vi "Create Sweep.vi"(6 "Post action (indexing priority)":T1=[enum."Do Nothing", enum."Wait", enum."Do Nothing", enum."Do Nothing"], 8 "error in (no error)":errorcluster, 9 "Scan parameters":T3=[{"DAQ Channel"=2, "Label"="\nscaledVsg1=", "Start"=0.14, "End"=-0.060000000000000005, "Step"=-0.060000000000000005, "Rate"=0.0, "VISA resource name"=""}, {"DAQ Channel"=2, "Label"="\nscaledVsg1=", "Start"=0.14, "End"=-0.060000000000000005, "Step"=-0.060000000000000005, "Rate"=0.0, "VISA resource name"=""}, {"DAQ Channel"=2, "Label"="\nscaledVsg1=", "Start"=0.14, "End"=-0.060000000000000005, "Step"=-0.060000000000000005, "Rate"=0.0, "VISA resource name"=""}, {"DAQ Channel"=3, "Label"="\nscaledVsg1=", "Start"=0.14, "End"=-0.060000000000000005, "Step"=-0.060000000000000005, "Rate"=0.0, "VISA resource name"=""}] {"Rate" format="%.2f"; "Step" format="%#_6p"; "End" format="%#_6p"; "Start" format="%#_6p"}, 10 "Scan control":T5=[{"Priority"=enum."Priority 1", "Scan name"=enum."DSA_Vamp"}, {"Priority"=enum."Priority 2", "Scan name"=enum."DSA_Vsg1"}, {"Priority"=enum."Priority 0", "Scan name"=enum."DSA_Vsg2"}, {"Priority"=enum."Priority 2", "Scan name"=enum."DSA_Vsg3"}], 11 "SweepControl":refnum<class "SweepControl.lvclass">) -> (0 "error out":errorcluster, 3 "SweepControl":refnum<class "SweepControl.lvclass">)   [LabVIEW 2016, in "SweepControl.lvclass"]
uses:
  SweepControl.lvclass
  Typedefs/ScanControl.ctl
  Typedefs/Cluster - ScanControl.ctl
  Typedefs/Enum - Priority.ctl
  Typedefs/Enum - Action.ctl
  Typedefs/ScanParamters.ctl
  Typedefs/Cluster - ScanParamters.ctl
  Typedefs/PostAction.ctl
  Typedefs/Enum - PostAction.ctl
  SweepControl.lvclass/SweepControl.ctl
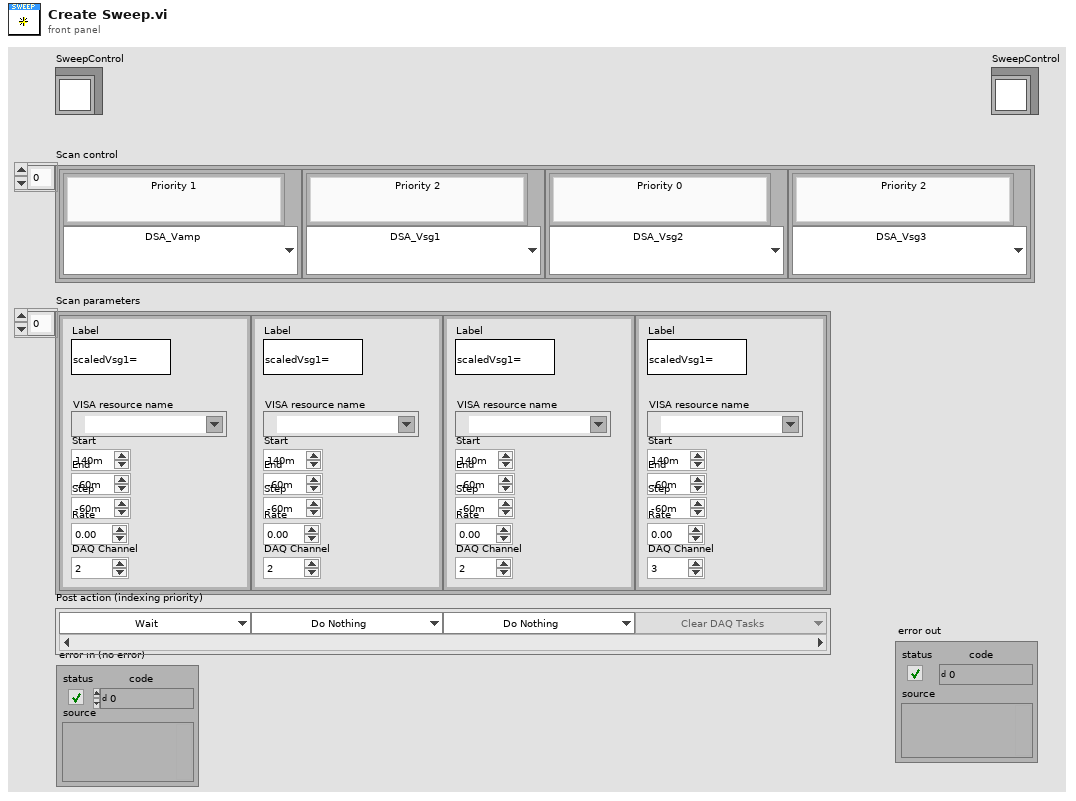
[diagram p1: front panel]
types:
  T1 = typedef "SweepControl.lvclass/PostAction.ctl" = T2[]
  T2 = typedef "SweepControl.lvclass/Enum - PostAction.ctl" = enum16{"Clear DAQ Tasks", "Check Temperature", "Wait", "Do Nothing"}
  T3 = typedef "SweepControl.lvclass/ScanParamters.ctl" = T4[]
  T4 = typedef "SweepControl.lvclass/Cluster - ScanParamters.ctl" = cluster{"DAQ Channel":i32, "Label":string, "Start":dbl, "End":dbl, "Step":dbl, "Rate":dbl, "VISA resource name":refnum<visa-resource-name>}
  T5 = typedef "SweepControl.lvclass/ScanControl.ctl" = T6[]
  T6 = typedef "SweepControl.lvclass/Cluster - ScanControl.ctl" = cluster{"Priority":T7, "Scan name":T8}
  T7 = typedef "SweepControl.lvclass/Enum - Priority.ctl" = enum16{"Priority 0", "Priority 1", "Priority 2", "Priority 3", "Priority 4", "Priority 5"}
  T8 = typedef "SweepControl.lvclass/Enum - Action.ctl" = enum16{"OFF", "DSA_Vamp", "DSA_freq", "DSA_Vsg1", "DSA_Vsg2", "DSA_Vsg3", "DAQ_Vbg", "B_Field", "Humidity", "Temp", "MW_freq1", "MW_freq2", "MW_amplitude1", "MW_amplitude2"}
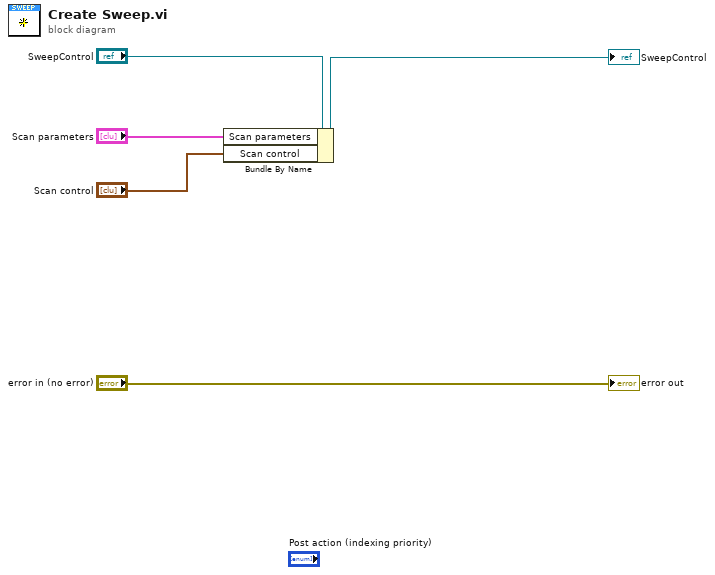
[diagram p0: block diagram]
diagram:
  n1 = Bundle By Name(cluster="SweepControl", "Scan parameters"="Scan parameters", "Scan control"="Scan control") -> (→"SweepControl":refnum<class "SweepControl.lvclass">)
  "error out" <- "error in (no error)"
